vi "Confirm Wire Reference.vi"(6 "Wire UID":i32, 8 "error in (no error)":errorcluster, 11 "Wire in":refnum<vi>) -> (0 "error out":errorcluster, 2 "Wire Refnum":refnum<vi>)   [LabVIEW 2018]
doc: "Gets the correct diagram reference to correct #Issue_004 where the asserts were being added incorrectly when inside a structure."
uses:
  <vilib>/Utility/error.llb/Error Cluster From Error Code.vi
  <vilib>/ErrorRing/Error Ring.xnode
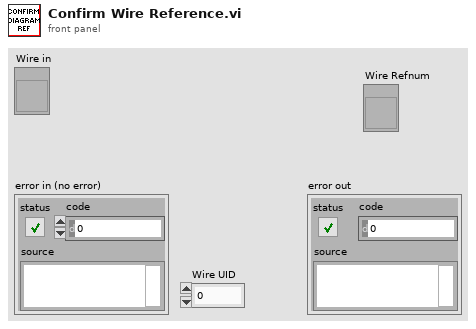
[diagram p1: front panel]
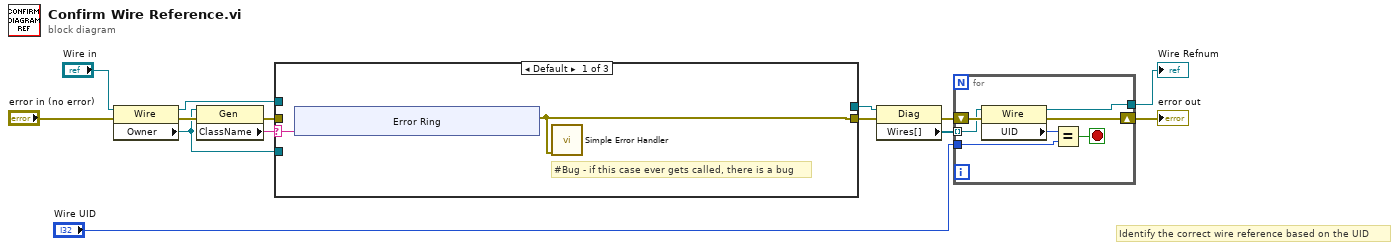
[diagram p0: block diagram]
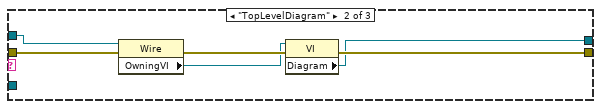
[diagram p2: hidden frame]
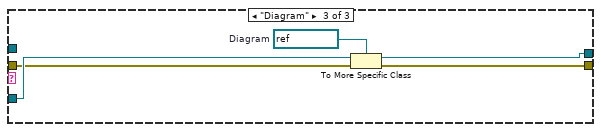
[diagram p3: hidden frame]
diagram:
  # "Identify the correct wire reference based on the UID"
  n1 = property class="Wire"(reference="Wire in", error in="error in (no error)") -> (reference out=w8:refnum<vi>, error out=w13:errorcluster, "Owner"=w10:refnum<vi>)
  n2 = property class="Gen"(reference=w10, error in=w13) -> (error out=w11:errorcluster, "ClassName"=w9:string)  [unwired: 1 out]
  n3 = case shown="Default" w9 {
    selector: w9 -> [w16 _ _]
    tunnel: [_ w24 w31] -> w4
    tunnel: w10 -> [_ _ w34]
    tunnel: [w15 w26 w30] -> w2
    tunnel: w11 -> [_ w28 w33]
    tunnel: w8 -> [_ w27 _]
    frame Default {
      # "#Bug - if this case ever gets called, there is a bug"
      n4 = xnode "Error Ring"("parameter 0"=w16) -> ("error out"=w15:errorcluster)
      n5 = call <vilib>:"Simple Error Handler.vi"("error in (no error)"=w15) -> ()  [unwired: 4 in, 5 out]
    }
    frame "TopLevelDiagram" {
      n6 = property class="Wire"(reference=w27, error in=w28) -> (error out=w29:errorcluster, "OwningVI"=w25:refnum<vi>)  [unwired: 1 out]
      n7 = property class="VI"(reference=w25, error in=w29) -> (error out=w26:errorcluster, "Diagram"=w24:refnum<vi>)  [unwired: 1 out]
    }
    frame "Diagram" {
      w32 = refnum<vi> refnum  # Diagram
      n8 = To More Specific Class(target class=w32, reference=w34, error in=w33) -> (specific class reference=w31:refnum<vi>, error out=w30:errorcluster)
    }
  }
  n9 = property class="Diag"(reference=w4, error in=w2) -> (error out=w7:errorcluster, "Wires[]"=w6:refnum<vi>[])  [unwired: 1 out]
  n10 = for {
    shift-right: [w40] -> w3
    shift-left: w7 -> [w41]
    tunnel: w6 -> [w39] mode=indexing
    tunnel: "Wire UID" -> [w37]
    tunnel: [w35] -> w1
    stop <- w36 stop-if-true
    n11 = property class="Wire"(reference=w39, error in=w41) -> (reference out=w35:refnum<vi>, error out=w40:errorcluster, "UID"=w38:i32)
    n12 = Equal?(x=w38, y=w37) -> (x = y?=w36:bool)
  }
  "error out" <- w3
  "Wire Refnum" <- w1
